vi "OwenPLC.vi"() -> ()   [LabVIEW 2020]
uses:
  <vilib>/NI/Modbus Library/API/Wrapper/Create Serial Master.vi
  <vilib>/NI/Modbus Library/API/Master/Modbus Master.lvclass
  <vilib>/NI/Modbus Library/API/Wrapper/API Main.lvlib
panel:
  out "register values":u16[](array[numeric])
  in  "OWEN PR200 monitoring_Dunin30_08_2021":enum32{"Settings", "Monitoring"}(tab)
  out "RS-485":errorcluster
  in  "VISA":refnum<visa-resource-name>="COM7"
  in  "baud rate":u32=115200
  in  "parity":u16(ring) items=["None", "Odd", "Even", "Mark", "Space"]
  in  "flow control":u16(ring) items=["None", "XON/XOFF", "RTS/CTS", "XON/XOFF & RTS/CTS", "DTR/DSR", "XON/XOFF & DTR/DSR"]
  in  "unit ID":u8=16
  in  "number of inputs":u16=8
  out "date":string
  out "time":string
  out "521":string
  out "520":string
  out "519":string
  out "518":string
  out "517":string
  out "516":string
  out "515":string
  out "514":string
  out "513":string
  out "DO 1":bool
  in  "?":bool
  out "register 512":u16
  out "register 513":u16
  out "register 514":u16
  out "register 515":u16
  out "register 516":u16
  out "register 517":u16
  out "register 518":u16
  out "register 519":u16
  out "DO 2":bool
  out "DO 3":bool
  out "DO 4":bool
  out "DO 5":bool
  out "DO 6":bool
  out "DO 8":bool
  out "DO 7":bool
  out "register 520":u16
  out "DO 9":bool
  out "register 521":u16
  out "DO 10":bool
  out "512":string
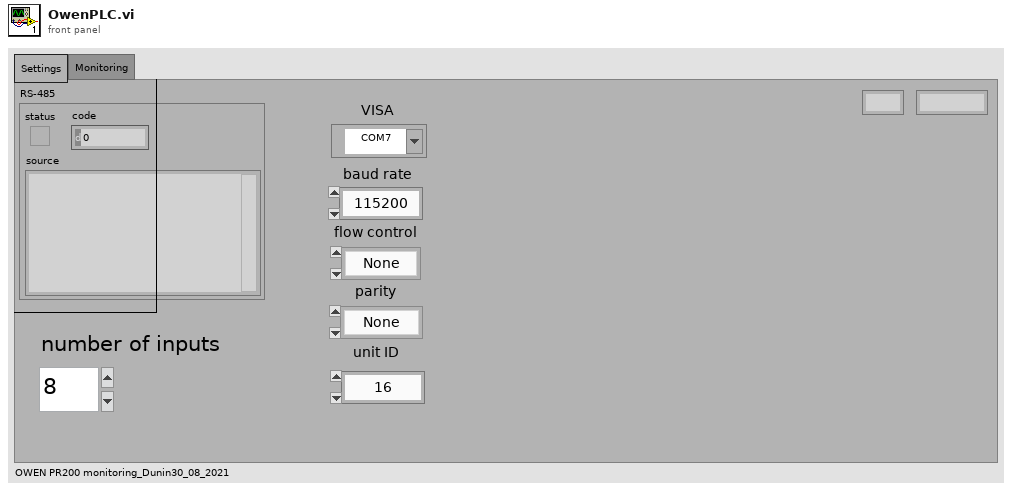
[diagram p1: front panel]
types:
  T1 = cluster{"register values[0]":u16, "register values[1]":u16, "register values[2]":u16, "register values[3]":u16, "register values[4]":u16, "register values[5]":u16, "register values[6]":u16, "register values[7]":u16, "register values[8]":u16}
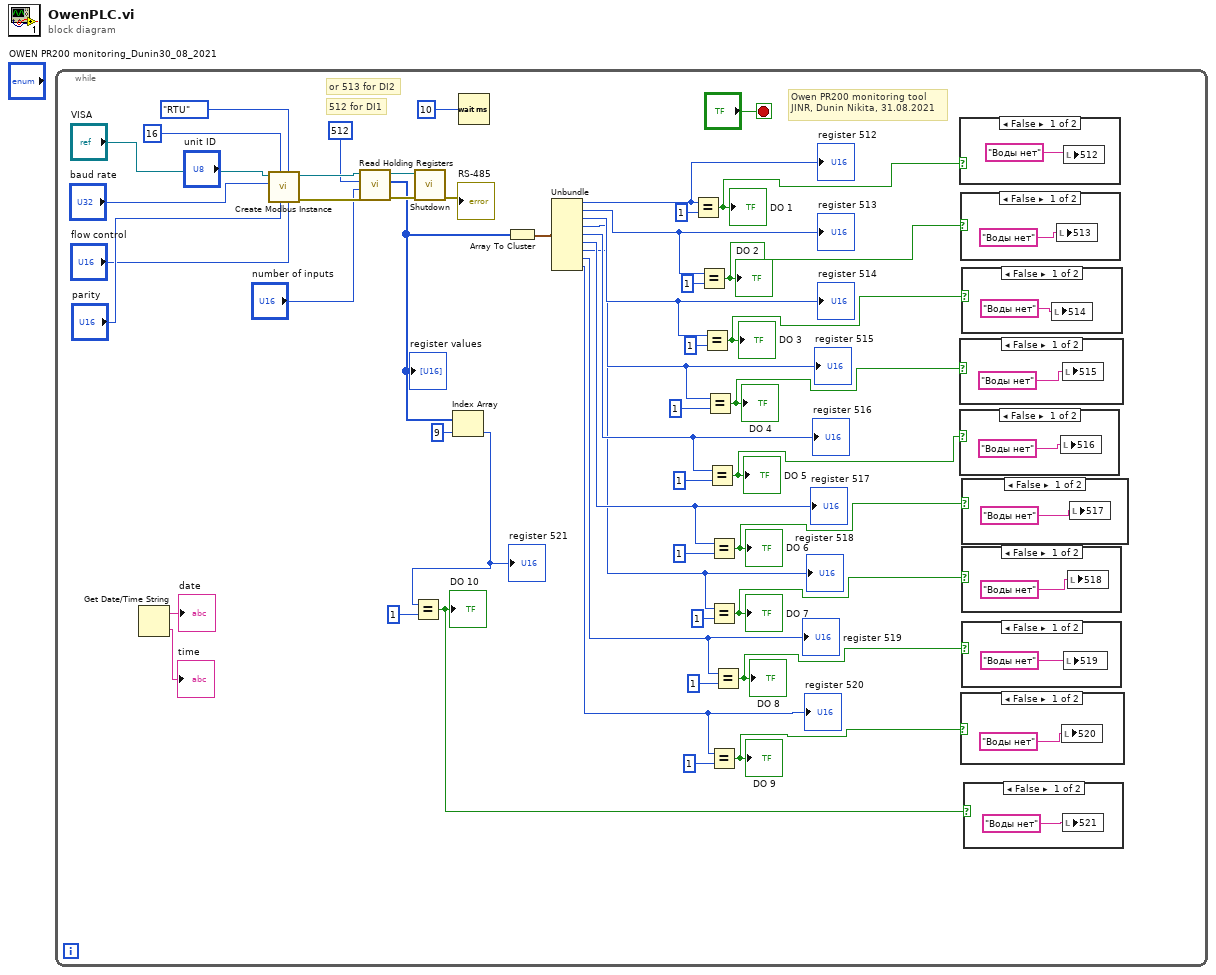
[diagram p0: block diagram]
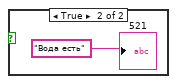
[diagram p2: hidden frame]
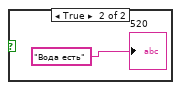
[diagram p3: hidden frame]
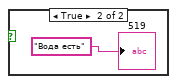
[diagram p4: hidden frame]
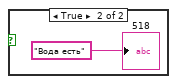
[diagram p5: hidden frame]
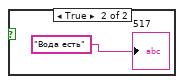
[diagram p6: hidden frame]
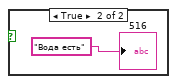
[diagram p7: hidden frame]
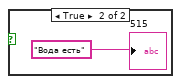
[diagram p8: hidden frame]
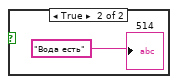
[diagram p9: hidden frame]
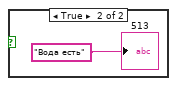
[diagram p10: hidden frame]
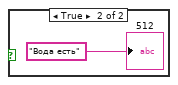
[diagram p11: hidden frame]
diagram:
  n1 = while {
    stop <- "?" stop-if-true
    # "Owen PR200 monitoring tool\nJINR, Dunin Nikita, 31.08.2021"
    # "512 for DI1"
    # "or 513 for DI2"
    n2 = Get Date/Time String() -> (date string=→"date":string, time string=→"time":string)  [unwired: 3 in]
    n3 = call-poly <vilib>:"Create Modbus Instance.vi"("flow control (none)"="flow control", "serial type"=enum16{"RTU", "ASCII"}."RTU", "parity (even)"="parity", "unit ID"=u8 16, "baud rate"="baud rate", "VISA resource name"="VISA") -> ("error out"=w44:errorcluster, "serial master instance"=w45:refnum<class "Modbus Master.lvclass">)  [unwired: 4 in]
    n4 = call-dynamic "Read Holding Registers.vi"("error in"=w44, "number of inputs"="number of inputs", "starting address"=u16 512, "Modbus master in"=w45) -> ("error out"=w40:errorcluster, "register values"=w16:u16[], "Modbus master out"=w41:refnum<class "Modbus Master.lvclass">)  [unwired: 5 in]
    "register values" <- w16
    n5 = call-dynamic "Shutdown.vi"("error in"=w40, "Modbus master in"=w41) -> ("error out"=→"RS-485":errorcluster)  [unwired: 9 in]
    n6 = Index Array(array=w16, index=9) -> (element=w13:u16)
    "register 521" <- w13
    n7 = Equal?(x=w13, y=1) -> (x = y?=w3:bool)
    "DO 10" <- w3
    n8 = Wait (ms)(milliseconds to wait=10) -> ()  [unwired: 1 out]
    n9 = Array To Cluster(array=w16) -> (cluster=w38:T1)
    n10 = Unbundle(w38) -> ("register values[0]"=w36:u16, "register values[1]"=w25:u16, "register values[2]"=w24:u16, "register values[3]"=w23:u16, "register values[4]"=w22:u16, "register values[5]"=w21:u16, "register values[6]"=w20:u16, "register values[7]"=w19:u16, "register values[8]"=w17:u16)
    "register 512" <- w36
    "register 513" <- w25
    "register 514" <- w24
    "register 515" <- w23
    "register 516" <- w22
    "register 517" <- w21
    "register 518" <- w20
    "register 519" <- w19
    "register 520" <- w17
    n11 = Equal?(x=w36, y=1) -> (x = y?=w12:bool)
    "DO 1" <- w12
    n12 = Equal?(x=w25, y=1) -> (x = y?=w11:bool)
    "DO 2" <- w11
    n13 = Equal?(x=w24, y=1) -> (x = y?=w10:bool)
    "DO 3" <- w10
    n14 = Equal?(x=w23, y=1) -> (x = y?=w9:bool)
    "DO 4" <- w9
    n15 = Equal?(x=w22, y=1) -> (x = y?=w8:bool)
    "DO 5" <- w8
    n16 = Equal?(x=w21, y=1) -> (x = y?=w7:bool)
    "DO 6" <- w7
    n17 = Equal?(x=w20, y=1) -> (x = y?=w6:bool)
    "DO 7" <- w6
    n18 = Equal?(x=w17, y=1) -> (x = y?=w4:bool)
    "DO 9" <- w4
    n19 = Equal?(x=w19, y=1) -> (x = y?=w5:bool)
    "DO 8" <- w5
    n20 = case shown="False" w12 {
      frame False {
        n21 = local write "512"("Воды нет") -> ()
      }
      frame True {
        "512" <- "Вода есть"
      }
    }
    n22 = case shown="False" w9 {
      frame False {
        n23 = local write "515"("Воды нет") -> ()
      }
      frame True {
        "515" <- "Вода есть"
      }
    }
    n24 = case shown="False" w8 {
      frame False {
        n25 = local write "516"("Воды нет") -> ()
      }
      frame True {
        "516" <- "Вода есть"
      }
    }
    n26 = case shown="False" w11 {
      frame False {
        n27 = local write "513"("Воды нет") -> ()
      }
      frame True {
        "513" <- "Вода есть"
      }
    }
    n28 = case shown="False" w4 {
      frame False {
        n29 = local write "520"("Воды нет") -> ()
      }
      frame True {
        "520" <- "Вода есть"
      }
    }
    n30 = case shown="False" w10 {
      frame False {
        n31 = local write "514"("Воды нет") -> ()
      }
      frame True {
        "514" <- "Вода есть"
      }
    }
    n32 = case shown="False" w7 {
      frame False {
        n33 = local write "517"("Воды нет") -> ()
      }
      frame True {
        "517" <- "Вода есть"
      }
    }
    n34 = case shown="False" w6 {
      frame False {
        n35 = local write "518"("Воды нет") -> ()
      }
      frame True {
        "518" <- "Вода есть"
      }
    }
    n36 = case shown="False" w5 {
      frame False {
        n37 = local write "519"("Воды нет") -> ()
      }
      frame True {
        "519" <- "Вода есть"
      }
    }
    n38 = case shown="False" w3 {
      frame False {
        n39 = local write "521"("Воды нет") -> ()
      }
      frame True {
        "521" <- "Вода есть"
      }
    }
  }
